vi "SerialCommunicationFast.vi"() -> ()   [LabVIEW 2011]
uses:
  <vilib>/FPGAPlugInAG/sbRIO-9636/niLvFpga_Open_sbRIO-9636.vi
  <vilib>/rvi/interface/common/dynamic/niFpgaDynamicAddResources.vi
  <vilib>/FPGAPlugInAG/Dynamic/niLvFpga_Run_Dynamic.vi
  <vilib>/Utility/error.llb/Error Cluster From Error Code.vi
  <vilib>/rvi/errors/niLvFpgaAdjustHostInterfaceError.vi
  <vilib>/FPGAPlugInAG/Dynamic/niLvFpga_Close_Dynamic.vi
  <vilib>/rvi/interface/nirviOpenFPGA/nirviOpenFPGA.xnode
  FPGA Bitfiles/TreadmillControl_FPGATarget_Exercise2_CF30559D.lvbitx
  FPGA/FPGA.vi
  <vilib>/rvi/interface/nirviMethod/nirviMethod.xnode
  <vilib>/rvi/interface/nirviCloseFPGA/nirviCloseFPGA.xnode
  <vilib>/FPGAPlugInAG/Dynamic/niLvFpga_ReadFifo_Dynamic.vi
  <vilib>/rvi/errors/niLvFpgaMergeErrorWithErrorCode.vi
panel:
  in  "RobotControl":cluster{"VlProfile":i16[], "VrProfile":i16[]}={"VlProfile"=[0, 0, 0, 0], "VrProfile"=[0, 0, 0, 0]}
  out "Voltage":cluster{"index":i32, "index":i32, "index":i32}(graph)
  in  "Sync":bool
  in  "LegGains":T1={"Kp"=1200, "Ki"=0, "Kd"=800, "Kaw"=0, "Kff"=0}
  out "Gyro":cluster{"index":i32, "index":i32, "index":i32}(graph)
  out "Accel":cluster{"index":i32, "index":i32, "index":i32}(graph)
  out "DataValues":i32[](array[numeric])
  in  "Format":i32[](array[numeric])=[4, 4, 4, 4, 4, 2, 2, 2, 2, 2, 2, 2, 2, 2, 2, 2]
  in  "EnableLog":bool
  in  "Timeout (ms)":i32
  in  "Number of Elements":u32=128
  out "DMA Queue Elements":u32(graph)
  out "PacketOut":u8[](array[numeric]) format="%02x"
  in  "PacketType":T2(ring)
  in  "Right":u16 format="%x"
  in  "Left":u16 format="%x"
  in  "Write":bool
  in  "Stop":bool
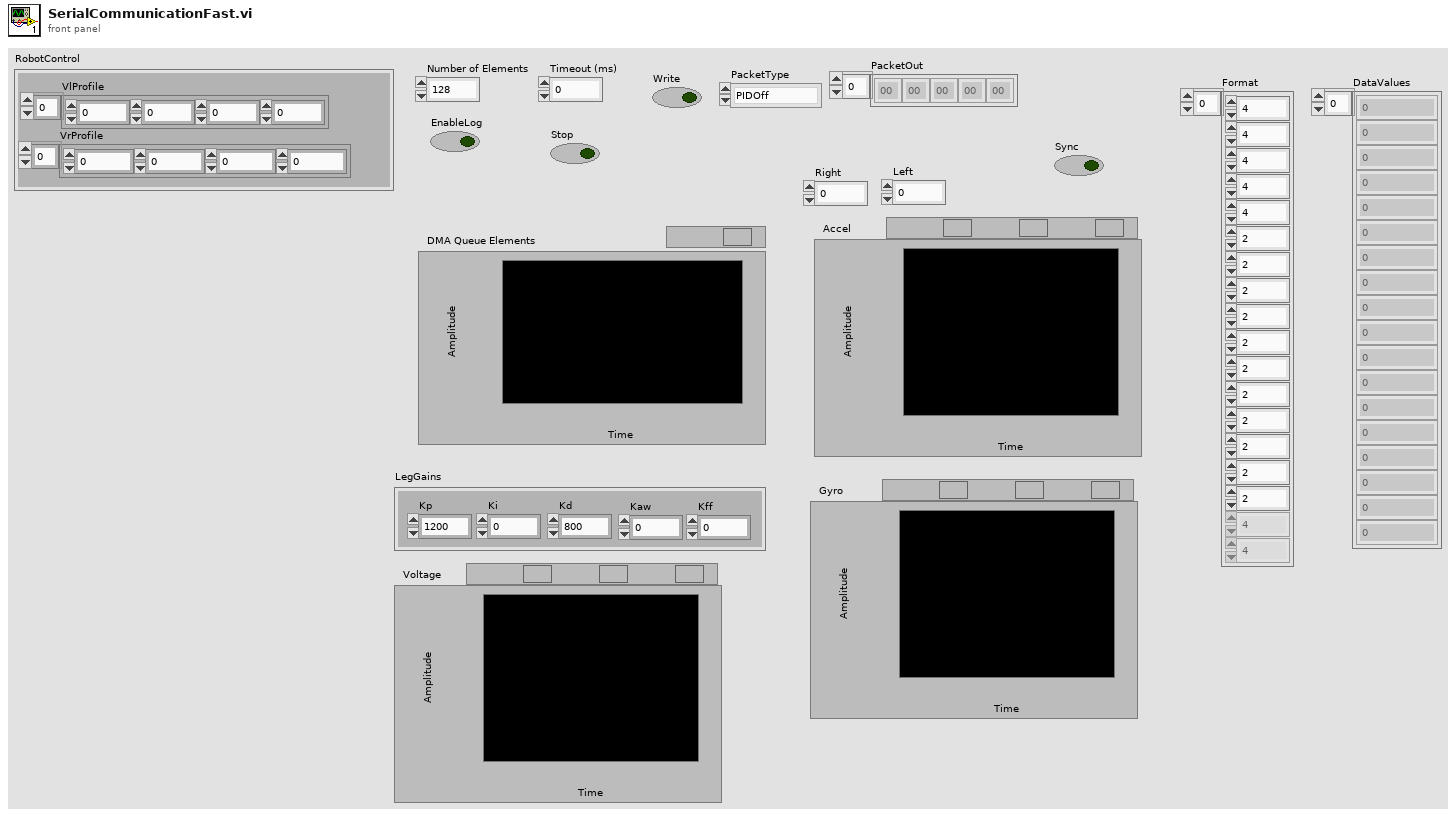
[diagram p1: front panel]
types:
  T1 = cluster{"Kp":u16, "Ki":u16, "Kd":u16, "Kaw":u16, "Kff":u16}
  T2 = enum16{"PIDOff", "PIDOn", "PIDSetProfile", "PIDSetGains", "ThrustOpenLoop"}
  T3 = enum16{"open", "replace", "create", "open or create", "replace or create", "replace or create with confirmation"}
  T4 = enum16{"big-endian, network order", "native, host order", "little-endian"}
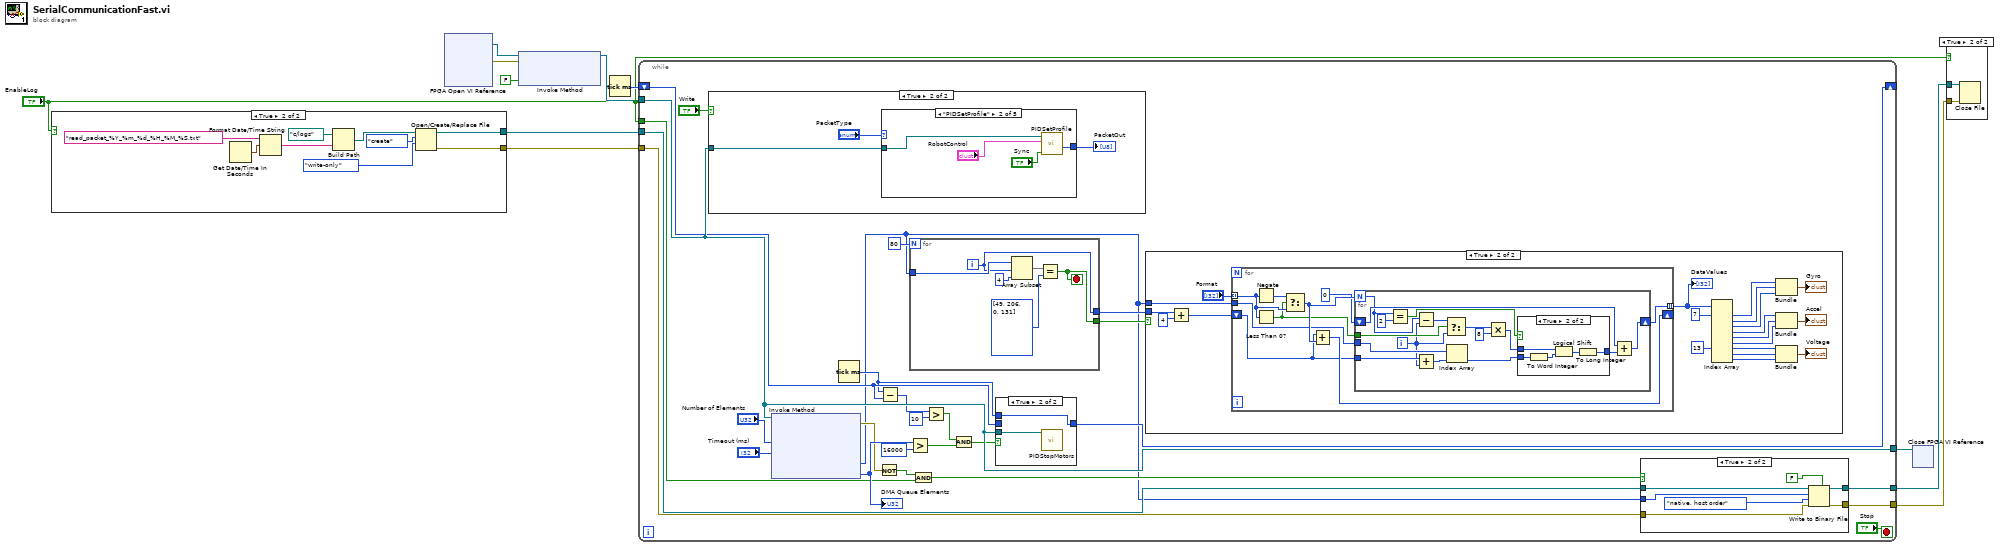
[diagram p0: block diagram]
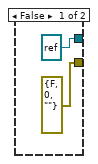
[diagram p3: hidden frame]
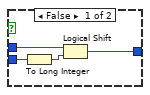
[diagram p5: hidden frame]
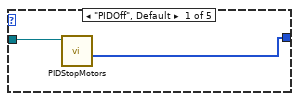
[diagram p9: hidden frame]
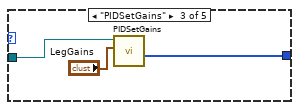
[diagram p10: hidden frame]
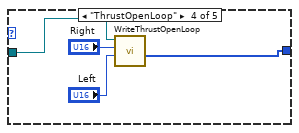
[diagram p11: hidden frame]
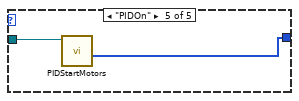
[diagram p12: hidden frame]
diagram:
  n1 = case shown="True" "EnableLog" {
    tunnel: [refnum<file> refnum ("refnum out") w15] -> w5
    tunnel: [errorcluster {"status"=FALSE, "code"=0, "source"=""} ("error out") w14] -> w4
    frame False {
    }
    frame True {
      n2 = Get Date/Time In Seconds() -> (seconds since 1Jan1904=w20:timestamp)
      n3 = Format Date/Time String(time format string (%c)="read_packet_%Y_%m_%d_%H_%M_%S.txt", seconds (now)=w20) -> (date/time string=w17:string)  [unwired: 1 in]
      n4 = Build Path(base path=path "c:/logs", name or relative path=w17) -> (appended path=w16:path)
      n5 = Open/Create/Replace File(file path (use dialog)=w16, operation (0:open)=T3."create", access (0:read/write)=enum16{"read/write", "read-only", "write-only"}."write-only") -> (refnum out=w15:refnum<file>, error out=w14:errorcluster)  [unwired: 3 in, 1 out]
    }
  }
  n6 = xnode "FPGA Open VI Reference"() -> ("FPGA VI Reference Out"=w6:refnum<k20>, "error out"=w7:errorcluster)  [unwired: 2 in]
  n7 = xnode "Invoke Method"("FPGA VI Reference In"=w6, "error in"=w7, "Wait Until Done (F)"=FALSE) -> ("FPGA VI Reference Out"=w9:refnum<k20>)  [unwired: 1 out]
  n8 = Tick Count (ms)() -> (millisecond timer value=w8:u32)
  n9 = while {
    tunnel: w9 -> [w43]
    tunnel: [w43] -> w10
    shift-right: [w42] -> _
    shift-left: w8 -> [w41]
    tunnel: "EnableLog" -> [w30]
    tunnel: w5 -> [w34]
    tunnel: w4 -> [w33]
    tunnel: [w32] -> w3
    tunnel: [w31] -> w2
    stop <- "Stop" stop-if-true
    n10 = case shown="True" "Write" {
      tunnel: w43 -> [_ w124]
      frame False {
      }
      frame True {
        n11 = case shown="\"PIDSetProfile\"" "PacketType" {
          tunnel: w124 -> [w126 w130 w133 w137 w139]
          tunnel: [w125 w129 w132 w134 w138] -> w122
          frame "PIDOff", Default {
            n12 = call "PIDStopMotors.vi"("Refnum in"=w126) -> ("PacketOut"=w125:u8[])  [unwired: 10 in]
          }
          frame "PIDSetProfile" {
            n13 = call "PIDSetProfile.vi"("Refnum in"=w130, "RobotControl"="RobotControl", "Sync"="Sync") -> ("PacketOut"=w129:u8[])  [unwired: 6 in]
          }
          frame "PIDSetGains" {
            n14 = call "PIDSetGains.vi"("Refnum in"=w133, "LegGains"="LegGains") -> ("PacketOut"=w132:u8[])  [unwired: 7 in]
          }
          frame "ThrustOpenLoop" {
            n15 = call "WriteThrustOpenLoop.vi"("Left"="Left", "Right"="Right", "Refnum in"=w137) -> ("PacketOut"=w134:u8[])  [unwired: 8 in]
          }
          frame "PIDOn" {
            n16 = call "PIDStartMotors.vi"("Refnum in"=w139) -> ("PacketOut"=w138:u8[])  [unwired: 10 in]
          }
        }
        "PacketOut" <- w122
      }
    }
    n17 = xnode "Invoke Method"("FPGA VI Reference In"=w43, "Number of Elements"="Number of Elements", "Timeout (ms)"="Timeout (ms)") -> ("error out"=w28:errorcluster, "Data"=w23:u8[], "Elements Remaining"=w45:u32)  [unwired: 1 in, 1 out]
    "DMA Queue Elements" <- w45
    n18 = Tick Count (ms)() -> (millisecond timer value=w35:u32)
    n19 = Not(x=w28) -> (.not. x?=w27:bool)
    n20 = Subtract(x=w35, y=w41) -> (x-y=w40:u32)
    n21 = for {
      N: 80 -> [_]
      tunnel: w23 -> [w109]
      tunnel: [w105] -> w25
      tunnel: [w104] -> w24
      i -> [w104]
      stop <- w105 stop-if-true
      n22 = Array Subset(array=w109, index=w104, length=4) -> (w107:u8[])
      n23 = Equal?(x=w107, y=u8[] [49, 206, 0, 131] ("Data")) -> (x = y?=w105:bool)
    }
    n24 = Greater?(x=w45, y=u32 16000) -> (0:w37:bool)
    n25 = And(x=w27, y=w30) -> (x .and. y?=w29:bool)
    n26 = Greater?(x=w40, y=u32 10) -> (0:w38:bool)
    n27 = And(x=w38, y=w37) -> (x .and. y?=w36:bool)
    n28 = case shown="True" w36 {
      tunnel: w43 -> [_ w121]
      tunnel: [w119 w120] -> w42
      tunnel: w41 -> [w119 _]
      tunnel: w35 -> [_ w120]
      frame False {
      }
      frame True {
        n29 = call "PIDStopMotors.vi"("Refnum in"=w121) -> ()  [unwired: 10 in, 1 out]
      }
    }
    n30 = case shown="True" w25 {
      tunnel: w24 -> [_ w69]
      tunnel: w23 -> [_ w65]
      frame False {
      }
      frame True {
        n31 = Add(x=w69, y=4 ("index")) -> (x+y=w66:i32)
        n32 = for {
          tunnel: "Format" -> [w78] mode=indexing
          shift-right: [w76] -> _
          shift-left: w66 -> [w72]
          tunnel: w65 -> [w74]
          tunnel: [w70] -> w64 mode=indexing
          n33 = Negate(x=w78) -> (-x=w77:i32)
          n34 = Less Than 0?(x=w78) -> (x < 0?=w73:bool)
          n35 = Select(t=w77, s=w73, f=w78) -> (s? t:f=w75:i32)
          n36 = Add(x=w72, y=w75) -> (x+y=w76:i32)
          n37 = for {
            N: w75 -> [w84]
            tunnel: w74 -> [w94]
            tunnel: w73 -> [w89]
            tunnel: w72 -> [w93]
            shift-right: [w90] -> w70
            shift-left: 0 ("index") -> [w91]
            i -> [w88]
            n38 = Equal?(x=w84, y=2) -> (x = y?=w82:bool)
            n39 = Subtract(x=w84, y=w88) -> (x-y=w87:i32)
            n40 = Add(x=w93, y=w88) -> (x+y=w92:i32)
            n41 = Select(t=w87, s=w89, f=w88) -> (s? t:f=w85:i32)
            n42 = Index Array(array=w94, index=w92) -> (element=w80:u8)
            n43 = Multiply(x=w85, y=8) -> (x*y=w81:i32)
            n44 = case shown="True" w82 {
              tunnel: w81 -> [w98 w102]
              tunnel: w80 -> [w97 w101]
              tunnel: [w95 w99] -> w79
              frame False {
                n45 = To Long Integer(number=w97) -> (32bit integer=w96:i32)
                n46 = Logical Shift(y=w98, x=w96) -> (x << y=w95:i32)
              }
              frame True {
                n47 = To Word Integer(number=w101) -> (16bit integer=w103:i16)
                n48 = Logical Shift(y=w102, x=w103) -> (x << y=w100:i16)
                n49 = To Long Integer(number=w100) -> (32bit integer=w99:i32)
              }
            }
            n50 = Add(x=w91, y=w79) -> (x+y=w90:i32)
          }
        }
        "DataValues" <- w64
        n51 = Index Array(array=w64, index #1=7 ("index"), index #7=13 ("index")) -> (element #1=w62:i32, element #2=w61:i32, element #3=w60:i32, element #4=w58:i32, element #5=w57:i32, element #6=w56:i32, element #7=w52:i32, element #8=w51:i32, element #9=w50:i32)  [unwired: 7 in]
        n52 = Bundle("index"=w62, "index"=w61, "index"=w60) -> (→"Gyro":cluster{"index":i32, "index":i32, "index":i32})  [unwired: 1 in]
        n53 = Bundle("index"=w58, "index"=w57, "index"=w56) -> (→"Accel":cluster{"index":i32, "index":i32, "index":i32})  [unwired: 1 in]
        n54 = Bundle("index"=w52, "index"=w51, "index"=w50) -> (→"Voltage":cluster{"index":i32, "index":i32, "index":i32})  [unwired: 1 in]
      }
    }
    n55 = case shown="True" w29 {
      tunnel: w34 -> [w111 w118]
      tunnel: w33 -> [w110 w117]
      tunnel: [w111 w116] -> w32
      tunnel: [w110 w115] -> w31
      tunnel: w23 -> [_ w114]
      frame False {
      }
      frame True {
        n56 = Write to Binary File(file (use dialog)=w118, data=w114, error in=w117, 5:FALSE ("prepend array or string size? (T)"), 9:T4."native, host order" ("byte order (0:big-endian, network order)")) -> (refnum out=w116:refnum<file>, error out=w115:errorcluster)  [unwired: 1 in, 1 out]
      }
    }
  }
  n57 = xnode "Close FPGA VI Reference"("FPGA VI Reference In"=w10) -> ()  [unwired: 1 in, 1 out]
  n58 = case shown="True" "EnableLog" {
    tunnel: w3 -> [_ w141]
    tunnel: w2 -> [_ w140]
    frame False {
    }
    frame True {
      n59 = Close File(refnum=w141, error in=w140) -> ()  [unwired: 2 out]
    }
  }
